vi "Lookup Primary Historian.vi"(8 "error in (no error)":errorcluster, 11 "Historian Module in":refnum<class "Historian Module.lvclass">) -> (0 "error out":errorcluster, 3 "Historian Module out":refnum<class "Historian Module.lvclass">)   [LabVIEW 2020, in "VolatusHistorian.lvlib" / "Historian Module.lvclass"]
uses:
  Historian Module.lvclass
  Historian Module.lvclass/Historian Module.ctl
  Volatus/Module/Module.lvclass
  VolatusConfig/VolatusConfig.lvlib
  VolatusConfig/VolatusConfigElement/VolatusConfigElement.lvclass
  VolatusConfig/Meta Type.ctl
  lv-cdm/CDM-Config/Config Filter/Config Lookup.lvclass
  lv-cdm/CDM-Config/Config Element/Config Element.lvclass
  VolatusConfig/Cluster/Cluster Config.lvclass
  C:/dev/lv20CE/relink/lv-volatus/VolatusConfig/VolatusConfigElement/VolatusConfigElement.lvclass
  C:/dev/lv20CE/relink/lv-volatus/VolatusConfig/Cluster/Cluster Config.lvclass
  C:/dev/lv20CE/relink/lv-volatus/Volatus/Module/Module.lvclass
  C:/dev/lv20CE/relink/lv-volatus/VolatusHistorian/Historian Module/Historian Module.lvclass
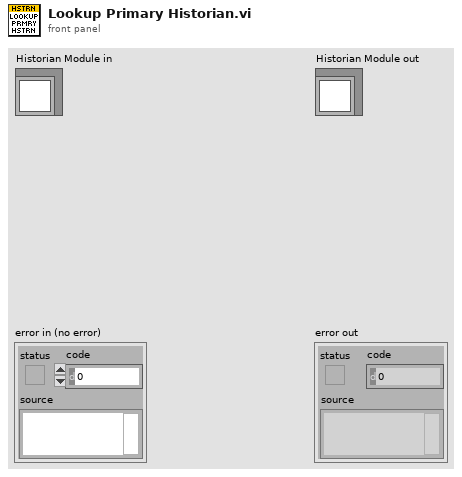
[diagram p1: front panel]
types:
  T1 = typedef "VolatusConfig.lvlib/Meta Type.ctl" = enum16{"UNKNOWN", "VL_System", "VL_Cluster", "VL_Node", "VL_Task", "VL_Group", "VL_Channel", "VL_Task_List", "VL_Scaling", "VL_Sensor", "VL_Sensor_List", "VL_Scale"}
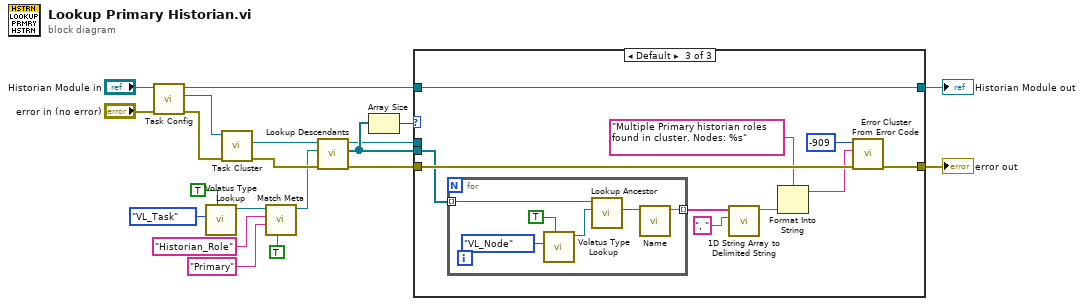
[diagram p0: block diagram]
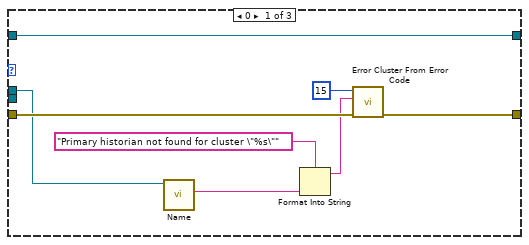
[diagram p2: hidden frame]
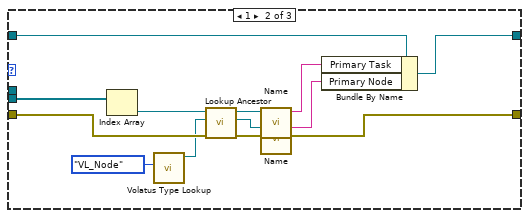
[diagram p3: hidden frame]
diagram:
  n1 = call "Task Config.vi"("error in (no error)"="error in (no error)", "Module in"="Historian Module in") -> ("error out"=w5:errorcluster, "Task Config"=w17:refnum<class "Task Config.lvclass">, "Module out"=w1:refnum<class "Historian Module.lvclass">)  [unwired: 7 in]
  n2 = call "Volatus Type Lookup.vi"("Don't Recurse Past Match (F)"=TRUE, "Meta Type"=Meta_Type."VL_Task") -> ("Config Lookup out"=w13:refnum<class "Config Lookup.lvclass">)  [unwired: 8 in, 1 out]
  n3 = call "Task Cluster.vi"("error in (no error)"=w5, "Task Config in"=w17) -> ("error out"=w20:errorcluster, "Cluster"=w16:refnum<class "Cluster Config.lvclass">)  [unwired: 7 in, 1 out]
  n4 = call "Match Meta.vi"("Exact Value (F)"=TRUE, "Value (Any)"="Primary" ("Name"), "Name"="Historian_Role", "Config Lookup (New)"=w13) -> ("Config Lookup out"=w9:refnum<class "Config Lookup.lvclass">)  [unwired: 6 in, 1 out]
  n5 = call "Lookup Descendants.vi"("error in (no error)"=w20, "Lookup"=w9, "VolatusConfigElement in"=w16) -> ("error out"=w6:errorcluster, "Descendants"=w7:refnum<class "Config Element.lvclass">[], "VolatusConfigElement out"=w3:refnum<class "Cluster Config.lvclass">)  [unwired: 6 in]
  n6 = Array Size(array=w7) -> (size(s)=w8:i32)
  n7 = case shown="Default" w8 {
    tunnel: w7 -> [_ w40 w49]
    tunnel: w6 -> [w28 w41 w51]
    tunnel: [w27 w30 w43] -> w4
    tunnel: w3 -> [w26 _ _]
    tunnel: [w21 w29 w42] -> w2
    tunnel: w1 -> [w21 w33 w42]
    frame 0 {
      n8 = call "Name.vi"("VolatusConfigElement in"=w26) -> ("Name"=w24:string)  [unwired: 8 in, 2 out]
      n9 = Format Into String(format string="Primary historian not found for cluster \"%s\"", w24) -> (resulting string=w23:string)  [unwired: 2 in, 1 out]
      n10 = call <vilib>:"Error Cluster From Error Code.vi"("error in (no error)"=w28, "error message (\"\")"=w23, "error code (0)"=15) -> ("error out"=w27:errorcluster)  [unwired: 6 in]
    }
    frame 1 {
      n11 = Index Array(array=w40) -> (element=w39:refnum<class "Config Element.lvclass">)  [unwired: 1 in]
      n12 = call "Volatus Type Lookup.vi"("Meta Type"=Meta_Type."VL_Node") -> ("Config Lookup out"=w37:refnum<class "Config Lookup.lvclass">)  [unwired: 9 in, 1 out]
      n13 = call "Lookup Ancestor.vi"("error in (no error)"=w41, "Lookup"=w37, "Config Element in"=w39) -> ("error out"=w34:errorcluster, "Ancestor"=w35:refnum<class "Config Element.lvclass">, "Config Element out"=w36:refnum<class "Config Element.lvclass">)  [unwired: 6 in]
      n14 = call "Name.vi"("Config Element in"=w36) -> ("Name"=w32:string)  [unwired: 9 in, 1 out]
      n15 = call "Name.vi"("error in (no error)"=w34, "Config Element in"=w35) -> ("error out"=w30:errorcluster, "Name"=w31:string)  [unwired: 8 in]
      n16 = Bundle By Name(cluster=w33, "Primary Task"=w32, "Primary Node"=w31) -> (w29:refnum<class "Historian Module.lvclass">)
    }
    frame Default {
      n17 = for {
        tunnel: w49 -> [w57] mode=indexing
        tunnel: [w52] -> w48 mode=indexing
        n18 = call "Volatus Type Lookup.vi"("Don't Recurse Past Match (F)"=TRUE, "Meta Type"=Meta_Type."VL_Node") -> ("Config Lookup out"=w54:refnum<class "Config Lookup.lvclass">)  [unwired: 8 in, 1 out]
        n19 = call "Lookup Ancestor.vi"("Lookup"=w54, "Config Element in"=w57) -> ("Ancestor"=w53:refnum<class "Config Element.lvclass">)  [unwired: 7 in, 2 out]
        n20 = call "Name.vi"("Config Element in"=w53) -> ("Name"=w52:string)  [unwired: 9 in, 1 out]
      }
      n21 = call <vilib>:"1D String Array to Delimited String.vi"("delimiter"=", ", "string array"=w48) -> ("delimited string"=w46:string)  [unwired: 9 in]
      n22 = Format Into String(format string="Multiple Primary historian roles found in cluster. Nodes: %s", w46) -> (resulting string=w44:string)  [unwired: 2 in, 1 out]
      n23 = call <vilib>:"Error Cluster From Error Code.vi"("error in (no error)"=w51, "error message (\"\")"=w44, "error code (0)"=-909) -> ("error out"=w43:errorcluster)  [unwired: 6 in]
    }
  }
  "error out" <- w4
  "Historian Module out" <- w2
